vi "BK Precision 9200 Series Run List Program.vi"() -> ()   [LabVIEW 2021]
doc: "This example demonstrates how to run a list program."
uses:
  <instrlib>/BK Precision 9200 Series/BK Precision 9200 Series.lvlib
panel:
  out "Actual Power Level (W)":dbl format="%.4g"
  out "Actual Voltage Level (V)":dbl format="%.4g"
  out "Actual Current Level (A)":dbl format="%.4g"
  in  "Stop List Program":bool
  in  "List Number (0)":i32 min=0 max=9 format="%#_0f"
  in  "VISA resource name":refnum<visa-resource-name>
  # "(c) 2014 B&K Precision Corporation.  ALL RIGHTS RESERVED."
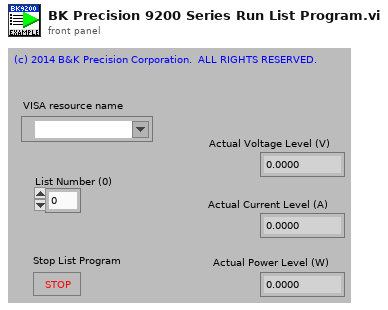
[diagram p1: front panel]
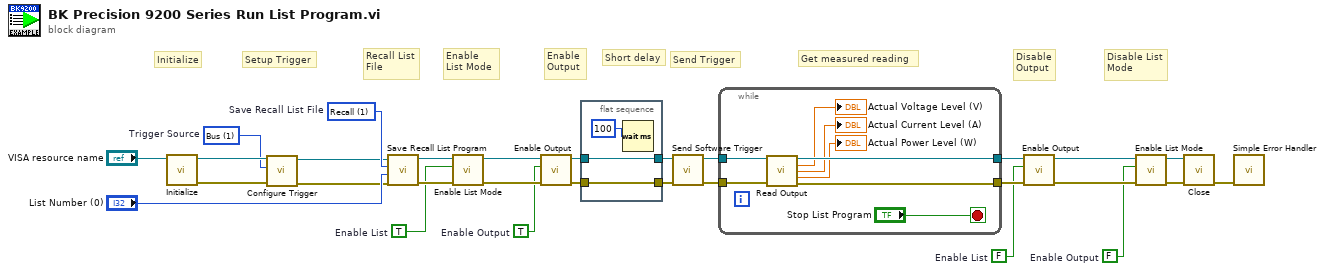
[diagram p0: block diagram]
diagram:
  w3 = 1 items=["Manual", "Bus"]  # Trigger Source
  w12 = FALSE  # Enable Output
  w1 = FALSE  # Enable List
  w2 = TRUE  # Enable Output
  w13 = TRUE  # Enable List
  w27 = u16 1 items=["Save", "Recall"]  # Save Recall List File
  # "Short delay"
  # "Setup Trigger"
  # "Initialize"
  # "Disable List\nMode"
  # "Disable\nOutput"
  # "Recall List\nFile"
  # "Enable\nList Mode"
  # "Enable\nOutput"
  # "Send Trigger"
  # "Get measured reading"
  n1 = call <instrlib>:"Initialize.vi"("VISA resource name"="VISA resource name") -> ("error out"=w8:errorcluster, "VISA resource name out"=w11:refnum<visa-resource-name>)  [unwired: 9 in]
  n2 = call <instrlib>:"Configure Trigger.vi"("error in (no error)"=w8, "Trigger Source (0:Manual)"=w3, "VISA resource name"=w11) -> ("error out"=w9:errorcluster, "VISA resource name out"=w10:refnum<visa-resource-name>)  [unwired: 7 in]
  n3 = call <instrlib>:"Save Recall List Program.vi"("error in (no error)"=w9, "List Number (0)"="List Number (0)", "Save Recall List File (0:Save)"=w27, "VISA resource name"=w10) -> ("error out"=w24:errorcluster, "VISA resource name out"=w25:refnum<visa-resource-name>)  [unwired: 6 in]
  n4 = call <instrlib>:"Enable List Mode.vi"("error in (no error)"=w24, "Enable List Mode (F: False)"=w13, "VISA resource name"=w25) -> ("error out"=w22:errorcluster, "VISA resource name out"=w23:refnum<visa-resource-name>)  [unwired: 7 in]
  n5 = call <instrlib>:"Enable Output.vi"("error in (no error)"=w22, "Enable Output (F: False)"=w2, "VISA resource name"=w23) -> ("error out"=w5:errorcluster, "VISA resource name out"=w6:refnum<visa-resource-name>)  [unwired: 7 in]
  n6 = flat-sequence {
    tunnel: [w32] -> w7
    tunnel: w6 -> [w32]
    tunnel: w5 -> [w31]
    tunnel: [w31] -> w4
    frame #0 {
      n7 = Wait (ms)(milliseconds to wait=100) -> ()  [unwired: 1 out]
    }
  }
  n8 = call <instrlib>:"Send Software Trigger.vi"("error in (no error)"=w4, "VISA resource name"=w7) -> ("error out"=w14:errorcluster, "VISA resource name out"=w17:refnum<visa-resource-name>)  [unwired: 8 in]
  n9 = while {
    tunnel: w17 -> [w39]
    tunnel: [w36] -> w16
    tunnel: [w37] -> w15
    tunnel: w14 -> [w38]
    stop <- "Stop List Program" stop-if-true
    n10 = call <instrlib>:"Read Output.vi"("VISA resource name"=w39, "error in (no error)"=w38) -> ("VISA resource name out"=w36:refnum<visa-resource-name>, "Actual Voltage Level (V)"=→"Actual Voltage Level (V)":dbl, "Actual Current Level (A)"=→"Actual Current Level (A)":dbl, "Actual Power Level (W)"=→"Actual Power Level (W)":dbl, "error out"=w37:errorcluster)  [unwired: 9 in]
  }
  n11 = call <instrlib>:"Enable Output.vi"("error in (no error)"=w15, "Enable Output (F: False)"=w1, "VISA resource name"=w16) -> ("error out"=w18:errorcluster, "VISA resource name out"=w19:refnum<visa-resource-name>)  [unwired: 7 in]
  n12 = call <instrlib>:"Enable List Mode.vi"("error in (no error)"=w18, "Enable List Mode (F: False)"=w12, "VISA resource name"=w19) -> ("error out"=w21:errorcluster, "VISA resource name out"=w20:refnum<visa-resource-name>)  [unwired: 7 in]
  n13 = call <instrlib>:"Close.vi"("error in (no error)"=w21, "VISA resource name"=w20) -> ("error out"=w28:errorcluster)  [unwired: 9 in]
  n14 = call <vilib>:"Simple Error Handler.vi"("error in (no error)"=w28) -> ()  [unwired: 4 in, 5 out]
